vi "A_2.vi"() -> ()   [LabVIEW 2020]
panel:
  in  "Loop delay [ms]":u32
  out "LED":bool
  in  "Discrimination level":dbl
  in  "Stop":bool
  out "Waveform Chart":cluster{"Dyscrimination level":dbl, dbl}(graph)
  in  "Noise amplitude":dbl
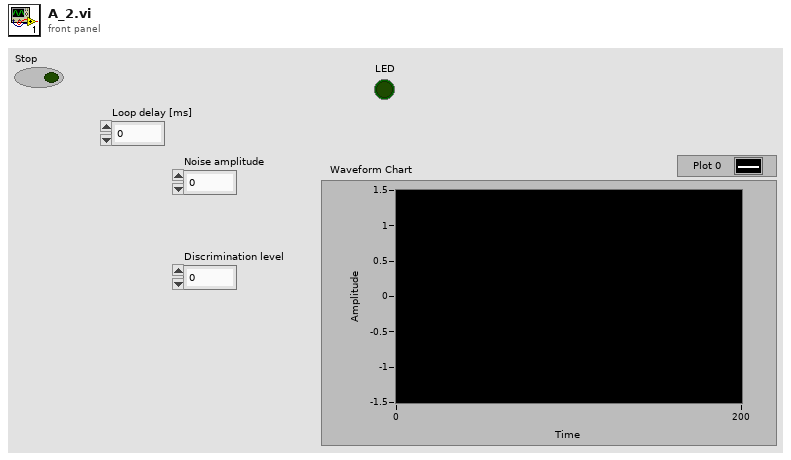
[diagram p1: front panel]
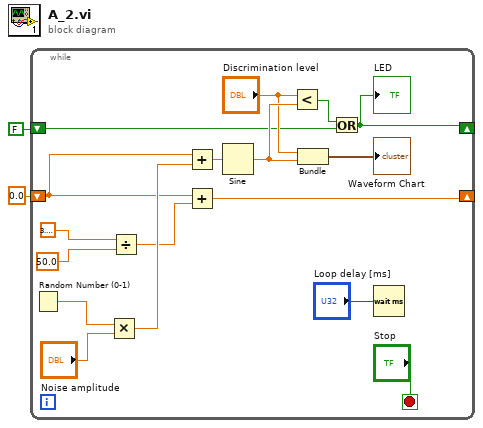
[diagram p0: block diagram]
diagram:
  n1 = while {
    shift-right: [w19] -> _
    shift-left: 0.0 -> [w15]
    shift-right: [w4] -> _
    shift-left: FALSE -> [w6]
    stop <- "Stop" stop-if-true
    n2 = Random Number (0-1)() -> (number: 0 to 1=w18:dbl)
    n3 = Multiply(x=w18, y="Noise amplitude") -> (x*y=w16:dbl)
    n4 = Divide(x=3.141592653589793, y=50.0 ("x")) -> (x/y=w12:dbl)
    n5 = Add(x=w15, y=w16) -> (x+y=w14:dbl)
    n6 = Add(x=w15, y=w12) -> (x+y=w19:dbl)
    n7 = Sine(x=w14) -> (sin(x)=w8:dbl)
    n8 = Less?(x="Discrimination level", y=w8) -> (x < y?=w5:bool)
    n9 = Bundle("Discrimination level"="Discrimination level", w8) -> (→"Waveform Chart":cluster{"Discrimination level":dbl, dbl})  [unwired: 1 in]
    n10 = Or(x=w5, y=w6) -> (x .or. y?=w4:bool)
    "LED" <- w4
    n11 = Wait (ms)(milliseconds to wait="Loop delay [ms]") -> ()  [unwired: 1 out]
  }
